vi "U8ToBoolean.vi"(1 "U8":u8) -> (0 "布尔":bool)   [LabVIEW 2012]
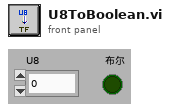
[diagram p1: front panel]
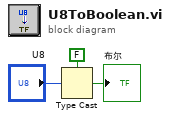
[diagram p0: block diagram]
diagram:
  n1 = Type Cast(type=FALSE ("布尔"), x="U8") -> (*(type *) &x=→"布尔":bool)
